vi "test_sensor_trigger.vi"() -> ()   [LabVIEW 2022 SP3]
uses:
  a32e15b2-a28c-4342-8085-9001f9b6d548.vi
  86df4578-fa6a-4ee3-a8c4-b72b936c298c.vi
  7a39ac04-e3a9-409e-b276-d0b84343f0e9.vi
  yaqc_labview/yaqc_labview_error_handler.vi
  yaqc-labview.lvlib
panel:
  out "Shape out":dbl[](array[numeric])
  out "Channel Units":string
  out "Measurement_id":i32
  out "Map Out":dbl[](array[numeric])
  out "Channel Names Out":string[](array[string])
  in  "Python path":path=path "C:/ProgramData/Anaconda3/envs/lv4/pythonw.exe"
  in  "Python version":string="3.8.0"
  in  "Python Module Path":path=path "C:/Users/kamey/work/labview/yaqc-labview/python/yaqc_labview.py"
  in  "Port":i32=39004
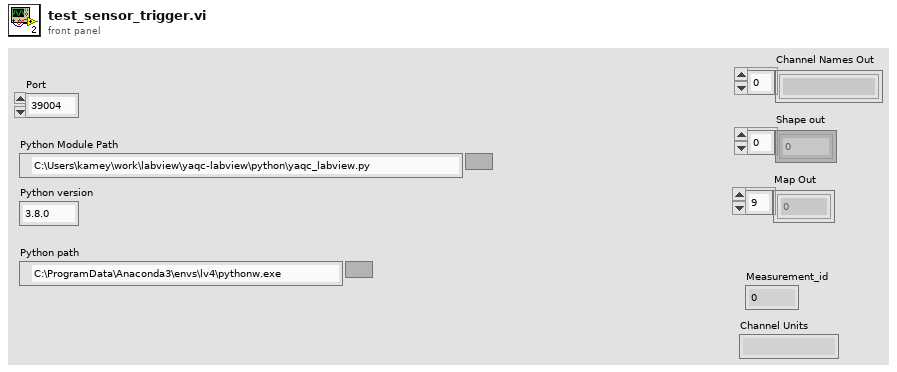
[diagram p1: front panel]
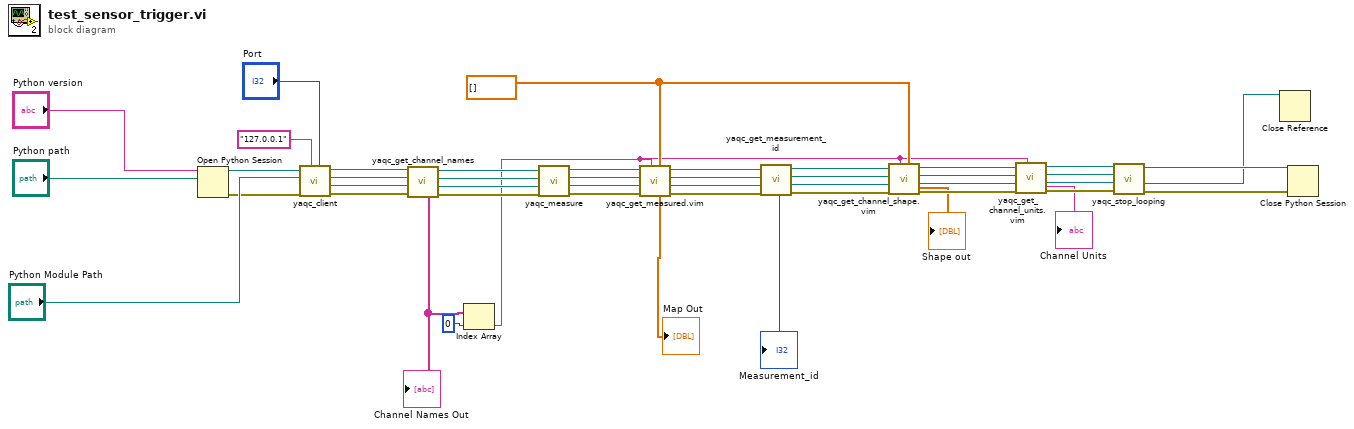
[diagram p0: block diagram]
diagram:
  w3 = dbl[] [] ("Map In")
  n1 = Open Python Session(python version="Python version", python path="Python path") -> (session out=w41:refnum<k35>, error out=w40:errorcluster)  [unwired: 1 in]
  n2 = call "yaqc_client.vi"("Port"="Port", "host ('127.0.0.1')"="127.0.0.1", "error in (no error)"=w40, "Python Module Path"="Python Module Path", "Python Session In"=w41) -> ("error out"=w39:errorcluster, "Yaqc Client"=w36:refnum<k38>, "Python Module Path Out"=w35:path, "Python Session Out"=w34:refnum<k35>)  [unwired: 3 in]
  n3 = call "yaqc_get_channel_names.vi"("error in (no error)"=w39, "Yaqc Client In"=w36, "Python Module Path In"=w35, "Python Session In"=w34) -> ("error out"=w30:errorcluster, "Yaqc Client Out"=w31:refnum<k38>, "Python Module Path Out"=w32:path, "Python Session Out"=w33:refnum<k35>, "Channel Names Out"=w37:string[])  [unwired: 3 in]
  "Channel Names Out" <- w37
  n4 = Index Array(array=w37, index=0) -> (element=w1:string)
  n5 = call "yaqc_measure.vi"("error in (no error)"=w30, "Yaqc Client In"=w31, "Python Module Path In"=w32, "Python Session In"=w33) -> ("error out"=w29:errorcluster, "Yaqc Client Out"=w22:refnum<k38>, "Python Module Path Out"=w23:path, "Python Session Out"=w24:refnum<k35>)  [unwired: 4 in]
  n6 = call "yaqc_get_measured.vim"("Array In"=w3, "Channel_name"=w1, "error in (no error)"=w29, "Yaqc Client In"=w22, "Python Module Path In"=w23, "Python Session In"=w24) -> ("error out"=w28:errorcluster, "Yaqc Client Out"=w27:refnum<k38>, "Python Module Path Out"=w26:path, "Python Session Out"=w25:refnum<k35>, "Array Out"=→"Map Out":dbl[])  [unwired: 1 in]
  n7 = call "yaqc_get_measurement_id.vi"("error in (no error)"=w28, "Yaqc Client In"=w27, "Python Module Path In"=w26, "Python Session In"=w25) -> ("error out"=w16:errorcluster, "Yaqc Client Out"=w8:refnum<k38>, "Python Module Path Out"=w9:path, "Python Session Out"=w10:refnum<k35>, "Measurement_id"=→"Measurement_id":i32)  [unwired: 3 in]
  n8 = call "yaqc_get_channel_shape.vim"("Shape in"=w3, "Channel_name"=w1, "error in (no error)"=w16, "Yaqc Client In"=w8, "Python Module Path In"=w9, "Python Session In"=w10) -> ("error out"=w15:errorcluster, "Yaqc Client Out"=w5:refnum<k38>, "Python Module Path Out"=w6:path, "Python Session Out"=w7:refnum<k35>, "Shape out"=→"Shape out":dbl[])  [unwired: 1 in]
  n9 = call "yaqc_get_channel_units.vim"("Channel_name"=w1, "error in (no error)"=w15, "Yaqc Client In"=w5, "Python Module Path In"=w6, "Python Session In"=w7) -> ("error out"=w14:errorcluster, "Yaqc Client Out"=w13:refnum<k38>, "Python Module Path Out"=w12:path, "Python Session Out"=w11:refnum<k35>, "Channel Units"=→"Channel Units":string)  [unwired: 2 in]
  n10 = call "yaqc_stop_looping.vi"("error in (no error)"=w14, "Yaqc Client In"=w13, "Python Module Path In"=w12, "Python Session In"=w11) -> ("error out"=w19:errorcluster, "Yaqc Client Out"=w17:refnum<k38>, "Python Session Out"=w18:refnum<k35>)  [unwired: 4 in, 1 out]
  n11 = Close Reference(reference=w17) -> ()  [unwired: 1 in, 1 out]
  n12 = Close Python Session(session in=w18, error in=w19) -> ()  [unwired: 1 out]
